vi "Reset Counter.vi"(2 "Reset":bool, 7 "Value":u16) -> (8 "Value":u16)   [LabVIEW 2011]
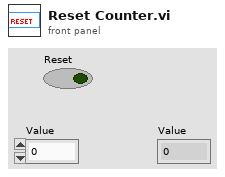
[diagram p1: front panel]
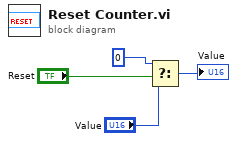
[diagram p0: block diagram]
diagram:
  n1 = Select(t=u16 0, s="Reset", f="Value") -> (s? t:f=→"Value":u16)
